vi "NoiseFilter.vi"(9 "loop":i32, 10 "lastCom":dbl, 11 "TemCom":dbl) -> (1 "VmicOut":dbl)   [LabVIEW 2020]
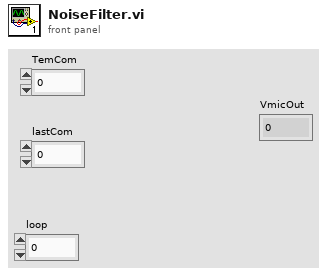
[diagram p1: front panel]
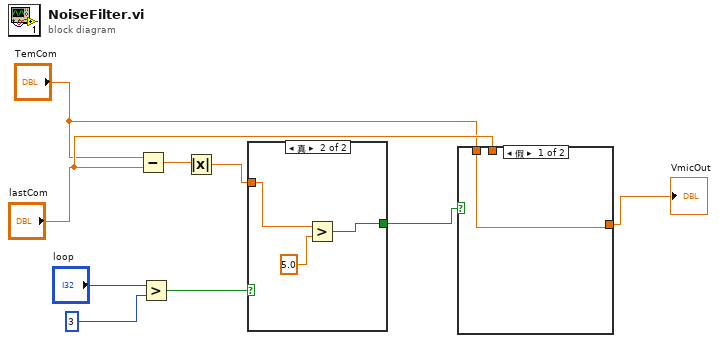
[diagram p0: block diagram]
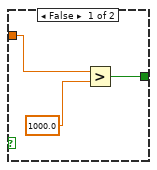
[diagram p3: hidden frame]
diagram:
  n1 = Subtract(x="TemCom", y="lastCom") -> (x-y=w9:dbl)
  n2 = Greater?(x="loop", y=3) -> (0:w6:bool)
  n3 = Absolute Value(x=w9) -> (abs(x)=w5:dbl)
  n4 = case shown="真" w6 {
    tunnel: w5 -> [w12 w15]
    tunnel: [w10 w13] -> w4
    frame False {
      n5 = Greater?(x=w12, y=1000.0) -> (0:w10:bool)
    }
    frame True {
      n6 = Greater?(x=w15, y=5.0) -> (0:w13:bool)
    }
  }
  n7 = case shown="假" w4 {
    tunnel: "lastCom" -> [_ w17]
    tunnel: "TemCom" -> [w16 _]
    tunnel: [w16 w17] -> w1
    frame False {
    }
    frame True {
    }
  }
  "VmicOut" <- w1
